vi "_keysight_write.vi"(1 "error in":errorcluster, 2 "command":string) -> (0 "error out":errorcluster)   [LabVIEW 2013]
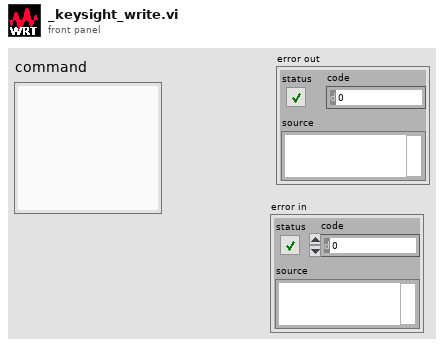
[diagram p1: front panel]
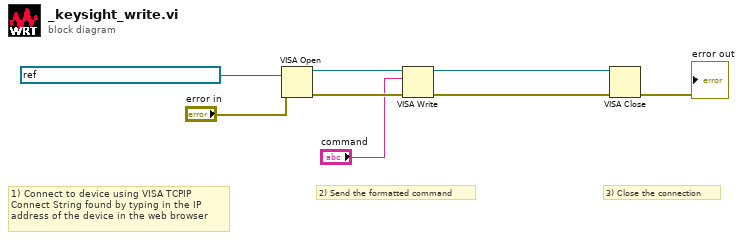
[diagram p0: block diagram]
diagram:
  # "3) Close the connection"
  # "1) Connect to device using VISA TCPIP Connect String found by typing in the IP address of the device in the web browser"
  # "2) Send the formatted command"
  n1 = VISA Open(error in (no error)="error in", VISA resource name=refnum<visa-resource-name> "TCPIP0::192.168.0.8::inst0::INSTR") -> (VISA resource name=w4:refnum<visa-resource-name>, error out=w5:errorcluster)  [unwired: 3 in]
  n2 = VISA Write(VISA resource name=w4, write buffer="command", error in (no error)=w5) -> (VISA resource name out=w6:refnum<visa-resource-name>, error out=w7:errorcluster)  [unwired: 1 out]
  n3 = VISA Close(VISA resource name=w6, error in (no error)=w7) -> (error out=→"error out":errorcluster)
